vi "audio-stim-play.vi"(3 "stop":bool, 11 "Stimulus List":dbl[][](array[numeric])=[[0.0, 3.0, 0.2, 1.0, 500.0], [1.0, 3.0, 0.2, 1.0, 500.0], [2.0, 3.0, 0.2, 1.0, 500.0], [3.0, 3.0, 0.2, 1.0, 1000.0], [4.0, 3.0, 0.2, 1.0, 500.0], [5.0, 3.0, 0.2, 1.0, 500.0], [6.0, 3.0, 0.2, 1.0, 1000.0], [7.0, 3.0, 0.2, 1.0, 1000.0], [8.0, 3.0, 0.2, 1.0, 1000.0], [9.0, 3.0, 0.2, 1.0, 500.0], [10.0, 3.0, 0.2, 1.0, 500.0], [11.0, 3.0, 0.2, 1.0, 1000.0], [12.0, 3.0, 0.2, 1.0, 1000.0], [13.0, 3.0, 0.2, 1.0, 1000.0], [14.0, 3.0, 0.2, 1.0, 1000.0], [15.0, 3.0, 0.2, 1.0, 1000.0], [16.0, 3.0, 0.2, 1.0, 500.0], [17.0, 3.0, 0.2, 1.0, 500.0], [18.0, 3.0, 0.2, 1.0, 500.0], [19.0, 3.0, 0.2, 1.0, 1000.0]]) -> ()   [LabVIEW 2013]
uses:
  <vilib>/DAQmx/write.llb/DAQmx Write (Digital U16 1Chan 1Samp).vi
  <vilib>/DAQmx/write.llb/DAQmx Write (Analog Wfm 1Chan NSamp).vi
  <vilib>/DAQmx/create/channels.llb/DAQmx Create Channel (AO-Voltage-Basic).vi
  <vilib>/DAQmx/create/channels.llb/DAQmx Create Channel (DO-Digital Output).vi
  <vilib>/DAQmx/miscellaneous.llb/DAQmx Fill In Error Info.vi
  <vilib>/DAQmx/configure/timing.llb/DAQmx Timing (Use Waveform).vi
panel:
  in  "Play Interval Jitter (s)":dbl=0.5
  in  "Play Interval (s)":dbl=1.0
  out "error out":errorcluster
  out "Playing":bool=TRUE caption="Playing stimulus"
  in  "DO Ports":tag="Dev1/port0:1" caption="DO Ports\n(\"browse\" and select two 8 bit ports)"
  in  "Sound AO Channel":tag="Dev1/ao0"
  out "Curr Param":dbl[](array[numeric])=[0.0, 3.0, 0.2, 1.0, 500.0] caption="Current (or Cued) Trial Parameters"
  in  "Sampling Rate":dbl=100000.0
  in  "Play":bool
  out "Current (or Cued) Waveform":waveform(dbl)(graph)={"t0"=timestamp(0 s since 1904-01-01), "dt"=1e-05, "Y"=array[19999 elements]}
  out "Waiting":bool=TRUE
  in  "Current (or Cued) Trial":i32(slide) min=0 max=20 scale=0.0..20.0
  # "Stim#, Stim Type, Duration, Amplitude, Param 1, Param 2, Param 3, Param 4"
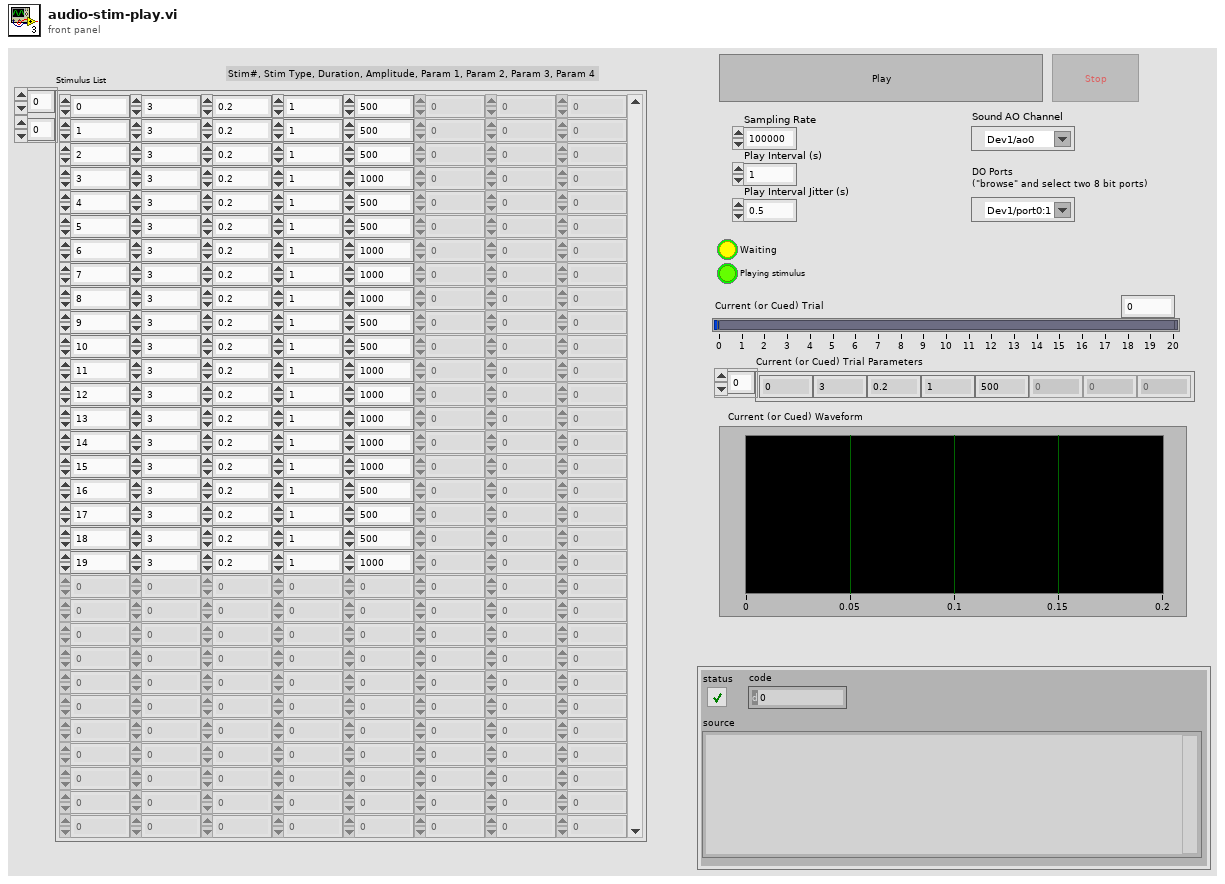
[diagram p1: front panel]
types:
  T1 = cluster{"Sampling Rate":dbl, "Value 3":dbl, dbl, "Value 2":dbl}
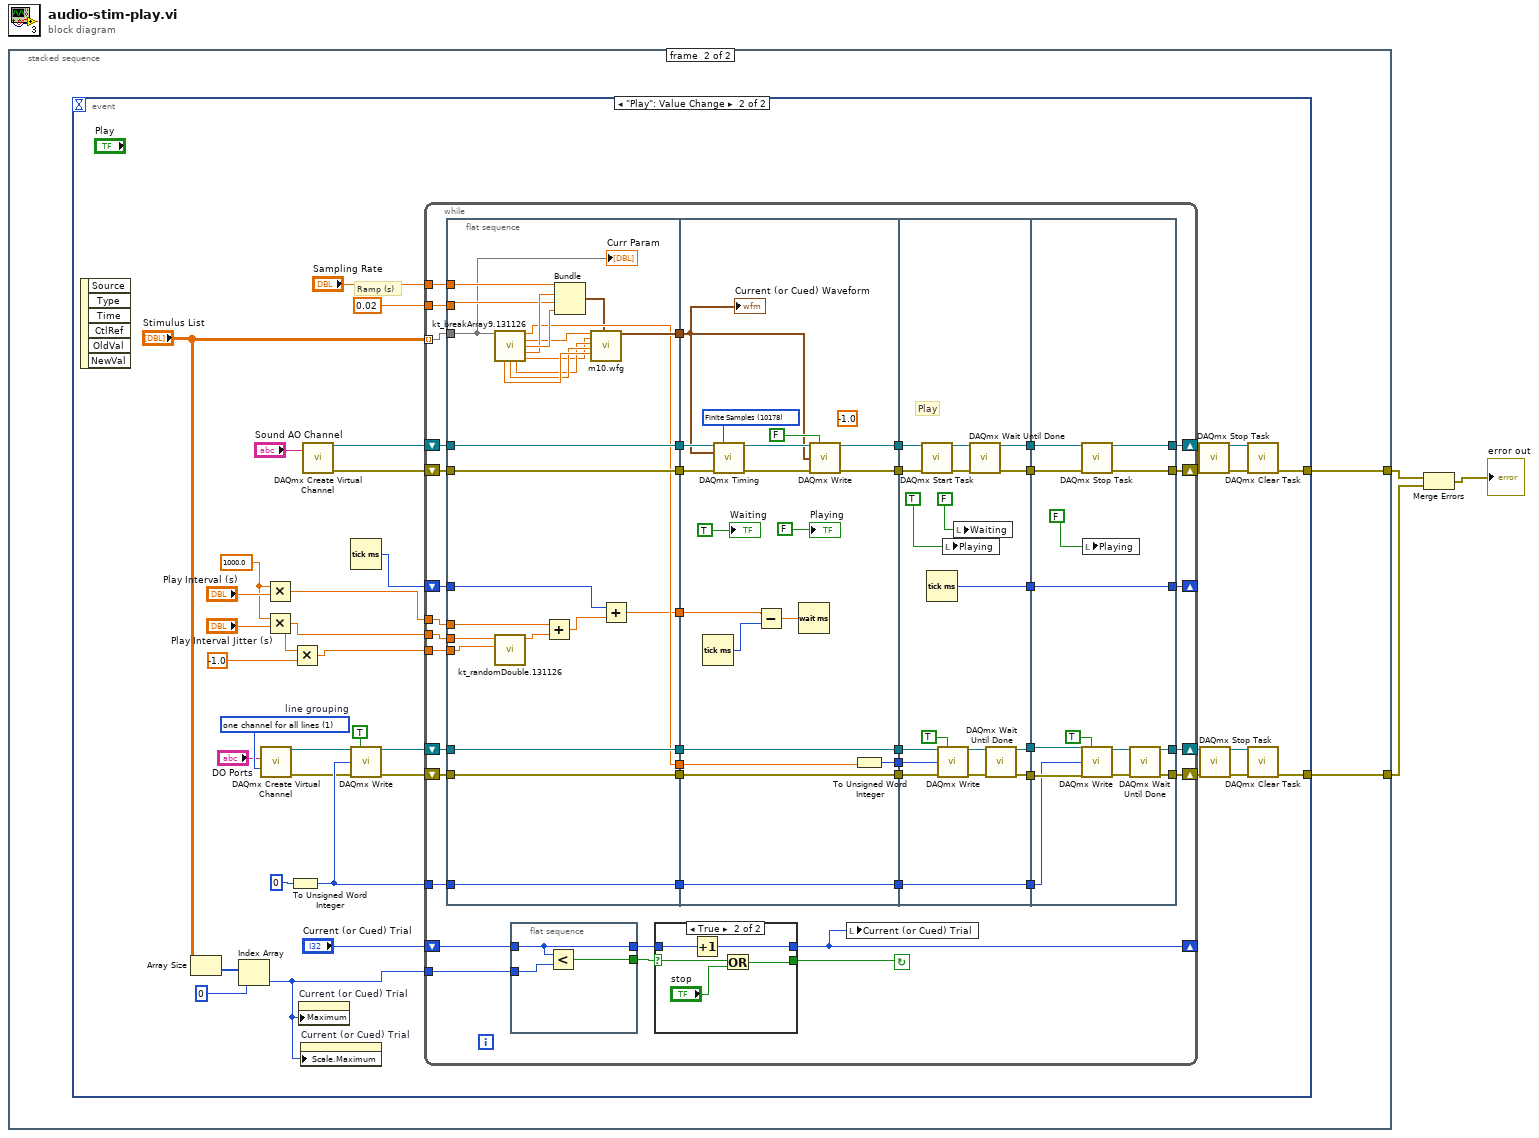
[diagram p0: block diagram]
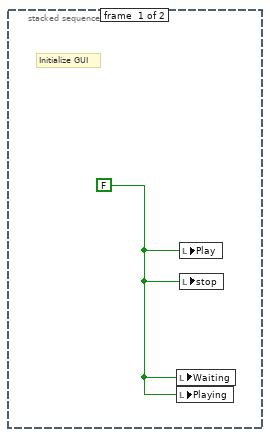
[diagram p2: hidden frame]
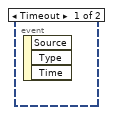
[diagram p3: hidden frame]
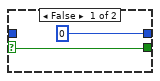
[diagram p4: hidden frame]
diagram:
  n1 = stacked-sequence {
    tunnel: [_ w6] -> w3
    tunnel: [_ w5] -> w2
    frame #0 {
      w4 = FALSE ("Play")
      # "Initialize GUI"
      n2 = local write "Waiting"(w4) -> ()
      n3 = local write "Playing"(w4) -> ()
      n4 = local write "Play"(w4) -> ()
      n5 = local write "stop"(w4) -> ()
    }
    frame #1 {
      n6 = event shown="[1] \"Play\": Value Change" {
        selector: _ -> [_ _]
        dyn-events: _ -> [_ _]
        timeout: _ -> [_ _]
        tunnel: [_ w19] -> w6
        tunnel: [_ w18] -> w5
        event Timeout {
          n7 = event-data() -> ()  [unwired: 1 in, 3 out]
        }
        event "Play": Value Change {
          w11 = 1000.0 ("y")
          w40 = 1 items=["one channel for each line", "one channel for all lines"]  # line grouping
          # "Ramp (s)"
          n8 = event-data() -> ()  [unwired: 1 in, 6 out]
          n9 = Array Size(array="Stimulus List") -> (size(s)=w38:i32[])
          n10 = Index Array(array=w38, index=0) -> (element=w22:i32)
          n11 = call-poly <vilib>:"DAQmx Create Virtual Channel.vi"("lines"="DO Ports", "line grouping"=w40) -> ("task out"=w16:refnum<k21>, "error out"=w15:errorcluster)  [unwired: 12 in]
          n12 = Multiply(x=w11, y="Play Interval (s)") -> (x*y=w10:dbl)
          n13 = Multiply(x=w11, y="Play Interval Jitter (s)") -> (x*y=w8:dbl)
          n14 = To Unsigned Word Integer(number=u16 0 ("data")) -> (unsigned 16bit integer=w23:u16)
          n15 = Multiply(x=w8, y=-1.0) -> (x*y=w9:dbl)
          n16 = property on="Current (or Cued) Trial" class="Slide (strict)"("Maximum"=w22) -> ()  [unwired: 2 in, 2 out]
          n17 = property on="Current (or Cued) Trial" class="Slide (strict)"("Scale.Maximum"=w22) -> ()  [unwired: 2 in, 2 out]
          n18 = call-poly <vilib>:"DAQmx Create Virtual Channel.vi"("physical channels"="Sound AO Channel") -> ("task out"=w21:refnum<k21>, "error out"=w20:errorcluster)  [unwired: 13 in]
          n19 = Tick Count (ms)() -> (millisecond timer value=w7:u32)
          n20 = call-poly <vilib>:"DAQmx Write.vi"("task/channels in"=w16, "auto start"=TRUE, "data"=w23, "error in"=w15) -> ("task out"=w27:refnum<k21>, "error out"=w26:errorcluster)  [unwired: 9 in, 1 out]
          n21 = while {
            tunnel: "Stimulus List" -> [w54] mode=indexing
            tunnel: "Sampling Rate" -> [w53]
            tunnel: 0.02 -> [w52]
            shift-right: [w84] -> w32
            shift-left: w21 -> [w82]
            shift-right: [w83] -> w31
            shift-left: w20 -> [w81]
            shift-right: [w71] -> w36
            shift-left: w27 -> [w80]
            shift-right: [w70] -> w35
            shift-left: w26 -> [w62]
            shift-right: [w65] -> _
            shift-left: "Current (or Cued) Trial" -> [w74]
            tunnel: w22 -> [w73]
            tunnel: w23 -> [w68]
            shift-right: [w49] -> _
            shift-left: w7 -> [w48]
            tunnel: w10 -> [w44]
            tunnel: w9 -> [w45]
            tunnel: w8 -> [w46]
            stop <- w63 continue-if-true
            n22 = flat-sequence {
              tunnel: w62 -> [w117]
              tunnel: w68 -> [w118]
              tunnel: w80 -> [w119]
              tunnel: w81 -> [w120]
              tunnel: w82 -> [w121]
              tunnel: [w121] -> w60
              tunnel: [w120] -> w59
              tunnel: [w119] -> w58
              tunnel: [w118] -> w57
              tunnel: [w117] -> w56
              tunnel: [w109] -> w55
              tunnel: w54 -> [w106]
              tunnel: w53 -> [w108]
              tunnel: w52 -> [w107]
              tunnel: [w105] -> w51
              tunnel: w48 -> [w103]
              tunnel: [w102] -> w47
              tunnel: w46 -> [w101]
              tunnel: w45 -> [w100]
              tunnel: w44 -> [w97]
              tunnel: [w130] -> w86
              tunnel: [w129] -> w85
              tunnel: [w139] -> w79
              tunnel: [w138] -> w72
              tunnel: [w137] -> w69
              tunnel: [w127] -> w61
              tunnel: w60 -> [w136]
              tunnel: w59 -> [w135]
              tunnel: w58 -> [w139]
              tunnel: w57 -> [w137]
              tunnel: w56 -> [w127]
              tunnel: w55 -> [w126]
              tunnel: w51 -> [w125]
              tunnel: w47 -> [w122]
              tunnel: w86 -> [w148]
              tunnel: w85 -> [w147]
              tunnel: w79 -> [w156]
              tunnel: [w150] -> w78
              tunnel: [w149] -> w77
              tunnel: [w153] -> w76
              tunnel: [w152] -> w75
              tunnel: w72 -> [w157]
              tunnel: w69 -> [w151]
              tunnel: [w151] -> w67
              tunnel: w61 -> [w142]
              tunnel: [w141] -> w50
              tunnel: [w160] -> w83
              tunnel: [w161] -> w84
              tunnel: w78 -> [w163]
              tunnel: w77 -> [w162]
              tunnel: w76 -> [w171]
              tunnel: w75 -> [w170]
              tunnel: [w166] -> w71
              tunnel: [w165] -> w70
              tunnel: w67 -> [w164]
              tunnel: w50 -> [w159]
              tunnel: [w159] -> w49
              frame #0 {
                n23 = call "kt_breakArray9.131126.vi"("Current (or Cued Trial Parameters)"=w106) -> ("Value 0"=w105:dbl, "Value 1"=w110:dbl, "Value 2"=w112:dbl, "Value 3"=w111:dbl, "Value 7"=w116:dbl, "Value 6"=w115:dbl, "Value 5"=w114:dbl, "Value 4"=w113:dbl)  [unwired: 6 in, 1 out]
                n24 = call "kt_randomDouble.131126.vi"("Min"=w100, "Max"=w101) -> ("Random"=w98:dbl)  [unwired: 9 in]
                n25 = Add(x=w97, y=w98) -> (x+y=w99:dbl)
                n26 = Bundle("Sampling Rate"=w108, "Value 3"=w111, w107, "Value 2"=w112) -> (w104:T1)  [unwired: 1 in]
                n27 = call "m10.wfg.vi"("Stimulus Type"=w110, "Param 0"=w113, "Param 1"=w114, "Param 2"=w115, "Param 3"=w116, "Waveform Properties"=w104) -> ("Waveform Out"=w109:waveform(dbl))  [unwired: 12 in, 1 out]
                n28 = Add(x=w103, y=w99) -> (x+y=w102:dbl)
                "Curr Param" <- w106
              }
              frame #1 {
                (unwired) -1.0 ("timeout")
                w134 = 10178 items=["Finite Samples"=10178, "Continuous Samples"=10123, "Hardware Timed Single Point"=12522] ("sample mode")
                n29 = Tick Count (ms)() -> (millisecond timer value=w123:u32)
                n30 = call-poly <vilib>:"DAQmx Timing.vi"("task/channels in"=w136, "sample mode"=w134, "waveform"=w126, "error in"=w135) -> ("task out"=w133:refnum<k21>, "error out"=w132:errorcluster)  [unwired: 10 in]
                n31 = Subtract(x=w122, y=w123) -> (x-y=w124:dbl)
                n32 = Wait (ms)(milliseconds to wait=w124) -> ()  [unwired: 1 out]
                n33 = call-poly <vilib>:"DAQmx Write.vi"("task/channels in"=w133, "auto start"=FALSE, "data"=w126, "error in"=w132) -> ("task out"=w130:refnum<k21>, "error out"=w129:errorcluster)  [unwired: 9 in, 1 out]
                n34 = To Unsigned Word Integer(number=w125) -> (unsigned 16bit integer=w138:u16)
                "Waiting" <- TRUE ("Playing Stimulus")
                "Playing" <- FALSE ("Playing Stimulus")
                "Current (or Cued) Waveform" <- w126
              }
              frame #2 {
                # "Play"
                n35 = call <vilib>:"DAQmx Start Task.vi"("task/channels in"=w148, "error in"=w147) -> ("task out"=w146:refnum<k21>, "error out"=w145:errorcluster)  [unwired: 12 in]
                n36 = Tick Count (ms)() -> (millisecond timer value=w141:u32)
                n37 = call-poly <vilib>:"DAQmx Write.vi"("task/channels in"=w156, "auto start"=TRUE, "data"=w157, "error in"=w142) -> ("task out"=w155:refnum<k21>, "error out"=w154:errorcluster)  [unwired: 9 in, 1 out]
                n38 = local write "Playing"(TRUE ("Playing Stimulus")) -> ()
                n39 = local write "Waiting"(FALSE ("Playing Stimulus")) -> ()
                n40 = call <vilib>:"DAQmx Wait Until Done.vi"("task/channels in"=w146, "error in"=w145) -> ("task out"=w150:refnum<k21>, "error out"=w149:errorcluster)  [unwired: 12 in]
                n41 = call <vilib>:"DAQmx Wait Until Done.vi"("task/channels in"=w155, "error in"=w154) -> ("task out"=w153:refnum<k21>, "error out"=w152:errorcluster)  [unwired: 12 in]
              }
              frame #3 {
                n42 = call <vilib>:"DAQmx Stop Task.vi"("task/channels in"=w163, "error in"=w162) -> ("task out"=w161:refnum<k21>, "error out"=w160:errorcluster)  [unwired: 12 in]
                n43 = call-poly <vilib>:"DAQmx Write.vi"("task/channels in"=w171, "auto start"=TRUE, "data"=w164, "error in"=w170) -> ("task out"=w168:refnum<k21>, "error out"=w167:errorcluster)  [unwired: 9 in, 1 out]
                n44 = local write "Playing"(FALSE ("Playing Stimulus")) -> ()
                n45 = call <vilib>:"DAQmx Wait Until Done.vi"("task/channels in"=w168, "error in"=w167) -> ("task out"=w166:refnum<k21>, "error out"=w165:errorcluster)  [unwired: 12 in]
              }
            }
            n46 = flat-sequence {
              tunnel: w74 -> [w94]
              tunnel: w73 -> [w96]
              tunnel: [w95] -> w64
              tunnel: [w94] -> w66
              frame #0 {
                n47 = Less?(x=w94, y=w96) -> (x < y?=w95:bool)
              }
            }
            n48 = case shown="True" w64 {
              selector: w64 -> [w87 w90]
              tunnel: w66 -> [_ w93]
              tunnel: [0 w92] -> w65
              tunnel: [w87 w91] -> w63
              frame False {
              }
              frame True {
                n49 = Increment(x=w93) -> (x+1=w92:i32)
                n50 = Or(x=w90, y="stop") -> (x .or. y?=w91:bool)
              }
            }
            n51 = local write "Current (or Cued) Trial"(w65) -> ()
          }
          n52 = call <vilib>:"DAQmx Stop Task.vi"("task/channels in"=w32, "error in"=w31) -> ("task out"=w30:refnum<k21>, "error out"=w29:errorcluster)  [unwired: 12 in]
          n53 = call <vilib>:"DAQmx Stop Task.vi"("task/channels in"=w36, "error in"=w35) -> ("task out"=w34:refnum<k21>, "error out"=w33:errorcluster)  [unwired: 12 in]
          n54 = call <vilib>:"DAQmx Clear Task.vi"("task in"=w30, "error in"=w29) -> ("error out"=w19:errorcluster)  [unwired: 13 in]
          n55 = call <vilib>:"DAQmx Clear Task.vi"("task in"=w34, "error in"=w33) -> ("error out"=w18:errorcluster)  [unwired: 13 in]
        }
      }
    }
  }
  n56 = Merge Errors(w3, w2) -> (→"error out":errorcluster)
